vi "Dynamic_3D_OBJ.vi"(0 "Color":u32(colorbox), 5 "Color 2":u32(colorbox), 9 "Color 3":u32(colorbox), 11 "Color 4":u32(colorbox)) -> (4 "SceneObject out":refnum<vi>, 6 "Child 3":refnum<vi>, 8 "Drawable":refnum<vi>, 10 "Child 2":refnum<vi>, 12 "Color 5":u32(colorbox), 13 "New Box Refnum":refnum<vi>, 14 "Child":refnum<vi>, 15 "Child 4":refnum<vi>)   [LabVIEW 2020]
uses:
  <vilib>/picture/3D Picture Control/Object/Create Object (name).vi
  <vilib>/picture/3D Picture Control/NI_3D Picture Control.lvlib
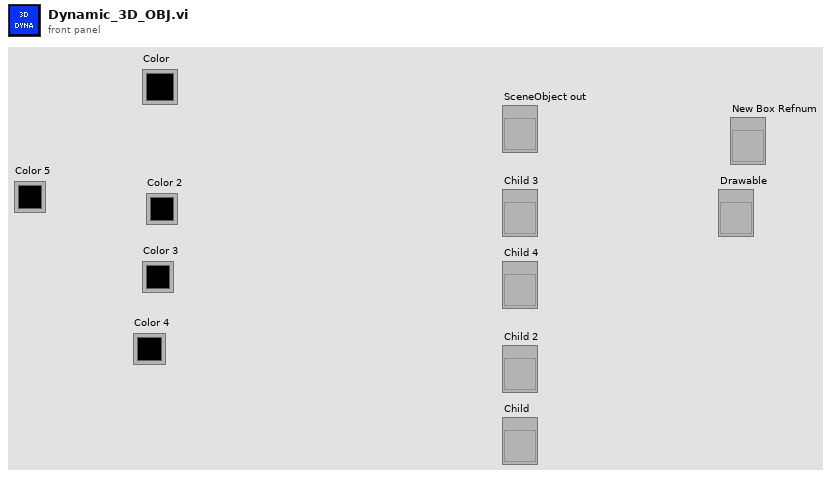
[diagram p1: front panel]
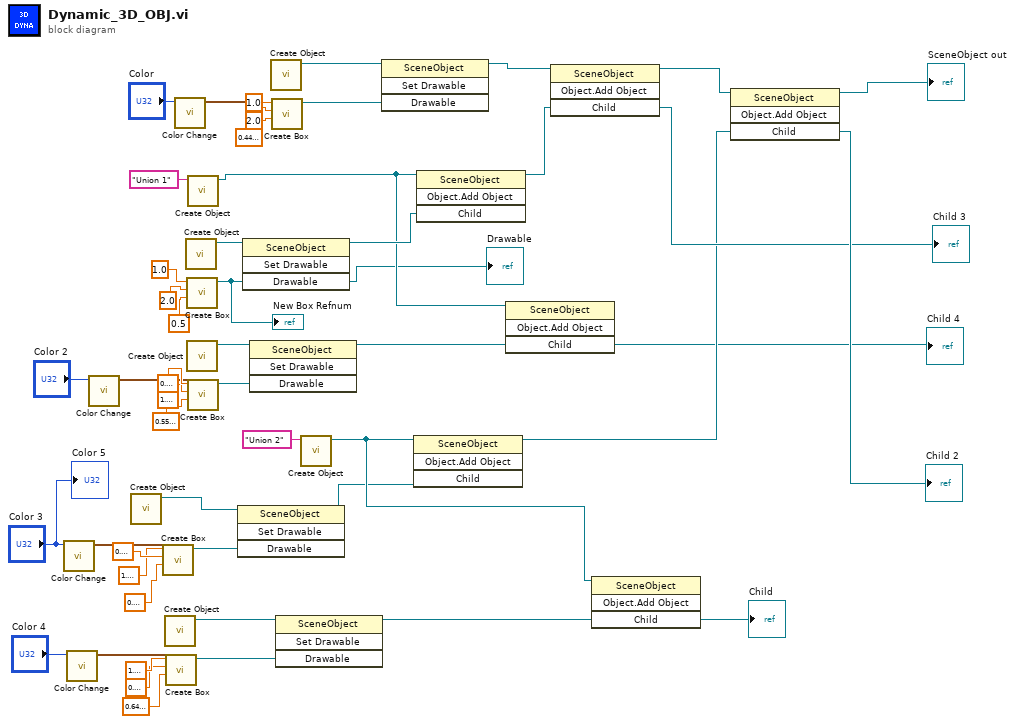
[diagram p0: block diagram]
diagram:
  n1 = call <vilib>:"Color Change.vi"("Color"="Color 3") -> ("RGBA"=w25:cluster{"R":sgl, "G":sgl, "B":sgl, "A":sgl})  [unwired: 10 in]
  n2 = call <vilib>:"Color Change.vi"("Color"="Color 4") -> ("RGBA"=w20:cluster{"R":sgl, "G":sgl, "B":sgl, "A":sgl})  [unwired: 10 in]
  n3 = call <vilib>:"Color Change.vi"("Color"="Color 2") -> ("RGBA"=w28:cluster{"R":sgl, "G":sgl, "B":sgl, "A":sgl})  [unwired: 10 in]
  n4 = call-poly <vilib>:"Create Object.vi"() -> ("Scene:New Object"=w27:refnum<vi>)  [unwired: 10 in, 1 out]
  n5 = call <vilib>:"Create Box.vi"("Color"=w25, "Length Z"=sgl 0.6, "Length Y"=sgl 0.8, "Length X"=sgl 1.8) -> ("New Box Refnum"=w26:refnum<vi>)  [unwired: 6 in, 1 out]
  n6 = call-poly <vilib>:"Create Object.vi"() -> ("Scene:New Object"=w23:refnum<vi>)  [unwired: 10 in, 1 out]
  n7 = call <vilib>:"Create Box.vi"("Color"=w20, "Length Z"=sgl 0.65, "Length Y"=sgl 0.7, "Length X"=sgl 1.7) -> ("New Box Refnum"=w22:refnum<vi>)  [unwired: 6 in, 1 out]
  n8 = call <vilib>:"Color Change.vi"("Color"="Color") -> ("RGBA"=w31:cluster{"R":sgl, "G":sgl, "B":sgl, "A":sgl})  [unwired: 10 in]
  n9 = call-poly <vilib>:"Create Object.vi"() -> ("Scene:New Object"=w12:refnum<vi>)  [unwired: 10 in, 1 out]
  n10 = call <vilib>:"Create Box.vi"("Length Z"=sgl 0.5, "Length Y"=sgl 2.0, "Length X"=sgl 1.0) -> ("New Box Refnum"=w2:refnum<vi>)  [unwired: 7 in, 1 out]
  "New Box Refnum" <- w2
  n11 = call-poly <vilib>:"Create Object.vi"() -> ("Scene:New Object"=w34:refnum<vi>)  [unwired: 10 in, 1 out]
  n12 = call-poly <vilib>:"Create Object.vi"("Name"="Union 1") -> ("Scene:New Object"=w8:refnum<vi>)  [unwired: 9 in, 1 out]
  n13 = call <vilib>:"Create Box.vi"("Color"=w28, "Length Z"=sgl 0.55, "Length Y"=sgl 1.9, "Length X"=sgl 0.9) -> ("New Box Refnum"=w33:refnum<vi>)  [unwired: 6 in, 1 out]
  n14 = invoke class="SceneObject" method="Set Drawable"(reference=w27, "Drawable"=w26) -> (reference out=w18:refnum<vi>)  [unwired: 2 in, 3 out]
  n15 = invoke class="SceneObject" method="Set Drawable"(reference=w12, "Drawable"=w2) -> (reference out=w10:refnum<vi>, "Drawable"=→"Drawable":refnum<vi>)  [unwired: 2 in, 2 out]
  n16 = invoke class="SceneObject" method="Set Drawable"(reference=w34, "Drawable"=w33) -> (reference out=w7:refnum<vi>)  [unwired: 2 in, 3 out]
  n17 = call-poly <vilib>:"Create Object.vi"() -> ("Scene:New Object"=w36:refnum<vi>)  [unwired: 10 in, 1 out]
  n18 = call <vilib>:"Create Box.vi"("Color"=w31, "Length Z"=sgl 0.45, "Length Y"=sgl 2.0, "Length X"=sgl 1.0) -> ("New Box Refnum"=w35:refnum<vi>)  [unwired: 6 in, 1 out]
  n19 = invoke class="SceneObject" method="Set Drawable"(reference=w23, "Drawable"=w22) -> (reference out=w17:refnum<vi>)  [unwired: 2 in, 3 out]
  n20 = call-poly <vilib>:"Create Object.vi"("Name"="Union 2") -> ("Scene:New Object"=w19:refnum<vi>)  [unwired: 9 in, 1 out]
  n21 = invoke class="SceneObject" method="Set Drawable"(reference=w36, "Drawable"=w35) -> (reference out=w32:refnum<vi>)  [unwired: 2 in, 3 out]
  n22 = invoke class="SceneObject" method="Object.Add Object"(reference=w19, "Child"=w18) -> (reference out=w16:refnum<vi>)  [unwired: 2 in, 3 out]
  n23 = invoke class="SceneObject" method="Object.Add Object"(reference=w8, "Child"=w10) -> (reference out=w9:refnum<vi>)  [unwired: 2 in, 3 out]
  n24 = invoke class="SceneObject" method="Object.Add Object"(reference=w8, "Child"=w7) -> ("Child"=→"Child 4":refnum<vi>)  [unwired: 2 in, 3 out]
  n25 = invoke class="SceneObject" method="Object.Add Object"(reference=w32, "Child"=w9) -> (reference out=w24:refnum<vi>, "Child"=→"Child 3":refnum<vi>)  [unwired: 2 in, 2 out]
  n26 = invoke class="SceneObject" method="Object.Add Object"(reference=w19, "Child"=w17) -> ("Child"=→"Child":refnum<vi>)  [unwired: 2 in, 3 out]
  n27 = invoke class="SceneObject" method="Object.Add Object"(reference=w24, "Child"=w16) -> (reference out=→"SceneObject out":refnum<vi>, "Child"=→"Child 2":refnum<vi>)  [unwired: 2 in, 2 out]
  "Color 5" <- "Color 3"
